vi "Save reference file -- subVI.vi"(8 "error in (no error)":errorcluster, 10 "Positions":dbl[](array[numeric]), 11 "Path":path) -> (0 "error out":errorcluster)   [LabVIEW 2020]
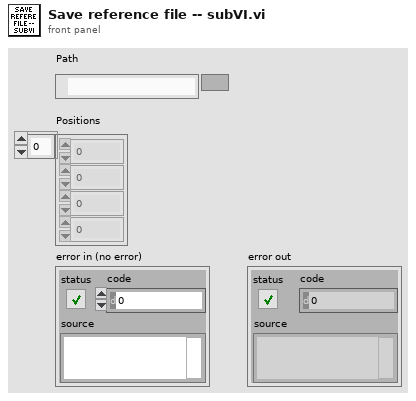
[diagram p1: front panel]
types:
  T1 = enum16{"open", "replace", "create", "open or create", "replace or create", "replace or create with confirmation"}
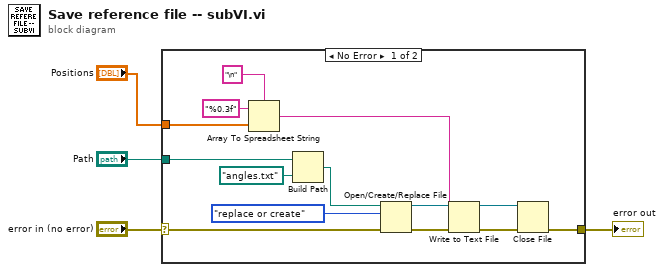
[diagram p0: block diagram]
diagram:
  n1 = case shown="No Error" "error in (no error)" {
    selector: "error in (no error)" -> [w13 w19]
    tunnel: "Positions" -> [w18 _]
    tunnel: "Path" -> [w16 _]
    tunnel: [w8 w19] -> w1
    frame No Error {
      n2 = Array To Spreadsheet String(delimiter (Tab)="\n", array=w18, 3:"%0.3f" ("format string")) -> (spreadsheet string=w7:string)
      n3 = Build Path(base path=w16, name or relative path=path "angles.txt") -> (appended path=w14:path)
      n4 = Open/Create/Replace File(file path (use dialog)=w14, error in=w13, operation (0:open)=T1."replace or create") -> (refnum out=w11:refnum<file>, error out=w12:errorcluster)  [unwired: 3 in, 1 out]
      n5 = Write to Text File(file (use dialog)=w11, text=w7, error in=w12) -> (refnum out=w9:refnum<file>, error out=w10:errorcluster)  [unwired: 1 in, 1 out]
      n6 = Close File(refnum=w9, error in=w10) -> (error out=w8:errorcluster)  [unwired: 1 out]
    }
    frame Error {
    }
  }
  "error out" <- w1
